vi "Main.vi"() -> ()   [LabVIEW 2016]
uses:
  User Events/User Event.lvclass
panel:
  in  "Stop":bool
  out "error out":errorcluster
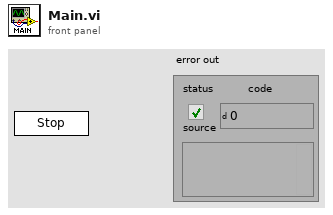
[diagram p1: front panel]
types:
  T1 = typedef "M1M3SupSimUserEvents.ctl" = cluster{"ILCResponse":refnum<user-event>, "StopUDPServer":refnum<user-event>}
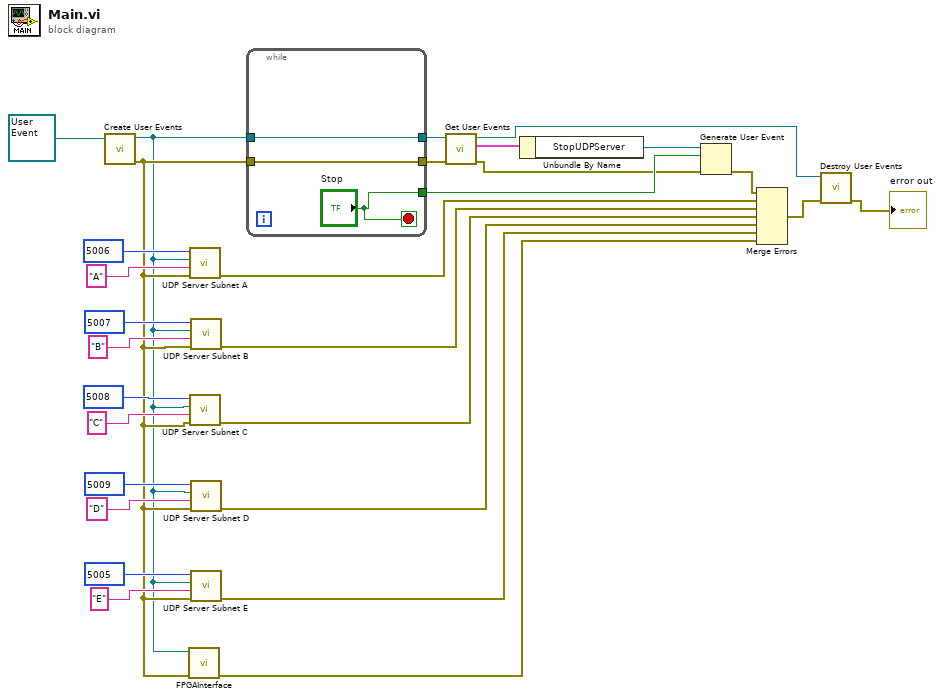
[diagram p0: block diagram]
diagram:
  n1 = call "Create User Events.vi"("User Event in"=refnum<class "User Event.lvclass"> refnum ("User Event.lvclass")) -> ("error out"=w3:errorcluster, "User Event out"=w2:refnum<class "User Event.lvclass">)  [unwired: 9 in]
  n2 = call "FPGAInterface.vi"("error in (no error)"=w3, "User Event in"=w2) -> ("error out"=w1:errorcluster)  [unwired: 9 in]
  n3 = call "UDP Server Subnet A.vi"("error in (no error)"=w3, "Subnet"="A", "User Event in"=w2, "UDP Port"=u16 5006) -> ("error out"=w21:errorcluster)  [unwired: 5 in, 2 out]
  n4 = call "UDP Server Subnet C.vi"("error in (no error)"=w3, "Subnet"="C", "User Event in"=w2, "UDP Port"=u16 5008) -> ("error out"=w6:errorcluster)  [unwired: 5 in, 2 out]
  n5 = call "UDP Server Subnet B.vi"("error in (no error)"=w3, "Subnet"="B", "User Event in"=w2, "UDP Port"=u16 5007) -> ("error out"=w7:errorcluster)  [unwired: 5 in, 2 out]
  n6 = call "UDP Server Subnet D.vi"("error in (no error)"=w3, "Subnet"="D", "User Event in"=w2, "UDP Port"=u16 5009) -> ("error out"=w5:errorcluster)  [unwired: 5 in, 2 out]
  n7 = call "UDP Server Subnet E.vi"("error in (no error)"=w3, "Subnet"="E", "User Event in"=w2, "UDP Port"=u16 5005) -> ("error out"=w4:errorcluster)  [unwired: 5 in, 2 out]
  n8 = while {
    tunnel: w2 -> [w32]
    tunnel: w3 -> [w31]
    tunnel: [w32] -> w26
    tunnel: [w31] -> w25
    tunnel: ["Stop"] -> w24
    stop <- "Stop" stop-if-true
  }
  n9 = call "Get User Events.vi"("error in (no error)"=w25, "User Event in"=w26) -> ("error out"=w23:errorcluster, "User Events"=w28:T1, "User Event out"=w22:refnum<class "User Event.lvclass">)  [unwired: 7 in]
  n10 = Unbundle By Name(w28) -> ("StopUDPServer"=w27:refnum<user-event>)
  n11 = Generate User Event(user event=w27, event data cluster=w24, error in=w23) -> (error out=w20:errorcluster)  [unwired: 1 in, 1 out]
  n12 = Merge Errors(w20, w21, w7, w6, w5, w4, w1) -> (w19:errorcluster)
  n13 = call "Destroy User Events.vi"("error in (no error)"=w19, "User Event in"=w22) -> ("error out"=→"error out":errorcluster)  [unwired: 8 in, 1 out]
